vi "Test MQTT-3.1.2-3.vi"(8 "error in (no error)":errorcluster) -> (0 "error out":errorcluster)   [LabVIEW 2013]
uses:
  <vilib>/LabVIEW Open Source Project/MQTT Control Packets/Control Packets/CONNECT/CONNECT.lvclass
  <vilib>/LabVIEW Open Source Project/MQTT Control Packets/Control Packets/ControlPacket/ControlPacket.lvclass
  <vilib>/addons/_JKI Toolkits/Caraya/classes/Test/Test.lvclass
  <vilib>/LabVIEW Open Source Project/MQTT Connection/MQTT_Connection/Connection/Connection.lvclass
  <vilib>/addons/_JKI Toolkits/Caraya/classes/Assert/Assert.lvclass
  <vilib>/addons/_JKI Toolkits/Caraya/classes/Assert/Assert Equal Value_Variant.vi
panel:
  out "timed out":bool
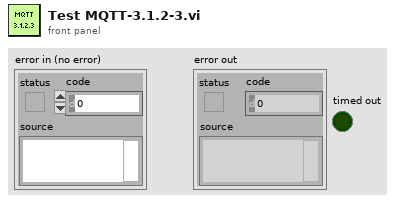
[diagram p1: front panel]
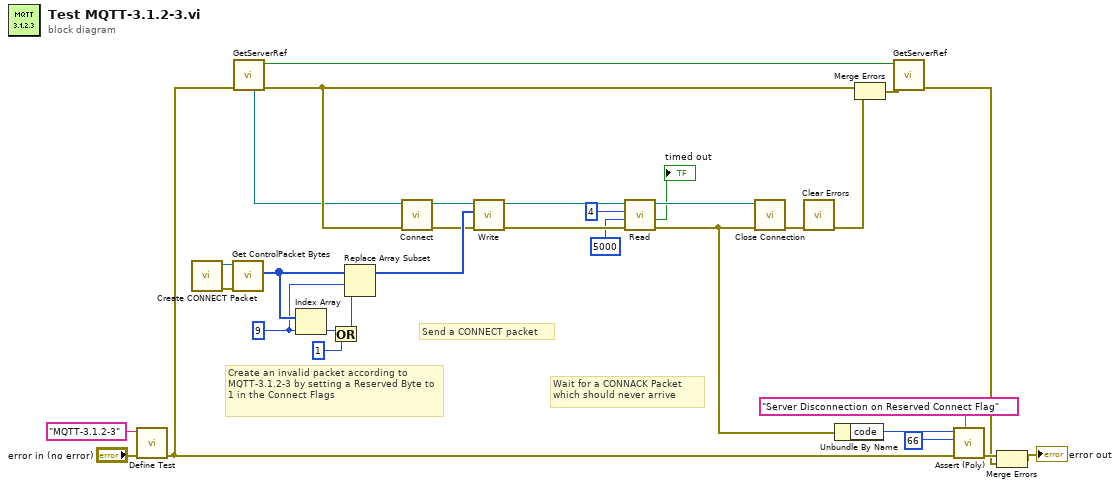
[diagram p0: block diagram]
diagram:
  w24 = 9 ("index")
  # "Wait for a CONNACK Packet\nwhich should never arrive"
  # "Create an invalid packet according to MQTT-3.1.2-3 by setting a Reserved Byte to 1 in the Connect Flags"
  # "Send a CONNECT packet"
  n1 = call <vilib>:"Define Test.vi"("error in (no error)"="error in (no error)", "Label (VI Title)"="MQTT-3.1.2-3") -> ("error out"=w7:errorcluster)  [unwired: 9 in]
  n2 = call <vilib>:"Create CONNECT Packet.vi"() -> ("error out"=w31:errorcluster, "CONNECT"=w32:refnum<class "CONNECT.lvclass">)  [unwired: 9 in, 1 out]
  n3 = call <vilib>:"Get ControlPacket Bytes.vi"("error in (no error)"=w31, "ControlPacket"=w32) -> ("Bytes Stream"=w26:u8[])  [unwired: 6 in, 3 out]
  n4 = call "GetServerRef.vi"("error in"=w7) -> ("error out"=w6:errorcluster, "Created"=w8:bool, "Connection Config"=w1:refnum<class "Connection.lvclass">)  [unwired: 7 in, 1 out]
  n5 = Index Array(array=w26, index=w24) -> (element=w28:u8)
  n6 = Or(x=w28, y=u8 1) -> (x .or. y?=w23:u8)
  n7 = Replace Array Subset(array=w26, new element=w23, index=w24) -> (w25:u8[])
  n8 = call <vilib>:"Connect.vi"("error in (no error)"=w6, "Connection in"=w1) -> ("error out"=w9:errorcluster, "Connection out"=w10:refnum<class "Connection.lvclass">)  [unwired: 8 in]
  n9 = call <vilib>:"Write.vi"("error in (no error)"=w9, "Bytes"=w25, "Connection in"=w10) -> ("error out"=w29:errorcluster, "Connection"=w30:refnum<class "Connection.lvclass">)  [unwired: 7 in]
  n10 = call <vilib>:"Read.vi"("error in (no error)"=w29, "timeout (2000 ms)"=5000 ("timeout ms (25000)"), "bytes to read (100)"=4 ("bytes to read"), "TCPConnection in"=w30) -> ("error out"=w12:errorcluster, "timed out"=→"timed out":bool, "TCPConnection out"=w22:refnum<class "Connection.lvclass">)  [unwired: 3 in, 2 out]
  n11 = call <vilib>:"Close Connection.vi"("error in (no error)"=w12, "Connection in"=w22) -> ("error out"=w16:errorcluster)  [unwired: 8 in, 1 out]
  n12 = call <vilib>:"Clear Errors.vi"("error in (no error)"=w16) -> ("error out"=w11:errorcluster)  [unwired: 6 in]
  n13 = Unbundle By Name(w12) -> ("code"=w3:i32)
  n14 = Merge Errors(w6, w11) -> (w4:errorcluster)
  n15 = call "GetServerRef.vi"("error in"=w4, "Destroy (F)"=w8) -> ("error out"=w5:errorcluster)  [unwired: 6 in, 3 out]
  n16 = call-poly <vilib>:"Assert (Poly).vi"("Label"="Server Disconnection on Reserved Connect Flag", "error in (no error)"=w7, "Y"=66 ("code"), "X"=w3) -> ("error out"=w20:errorcluster)  [unwired: 7 in]
  n17 = Merge Errors(w20, w5) -> (→"error out":errorcluster)
